vi "Configure SMU.vi"(5 "aperture time":dbl=0.001, 7 "Source Mode":enum16{"Voltage", "Current"}(ring), 8 "error in (no error)":errorcluster, 9 "Settings":T2 {"Sense" items=["Local"=1008, "Remote"=1009]}, 10 "Pins":string[](array[string]), 11 "Semiconductor Module Context":T3) -> (0 "error out":errorcluster)   [LabVIEW 2013]
uses:
  <vilib>/NI_TestStand_SemiconductorModule/NI_TestStand_Semiconductor_Module.lvlibp/PinMap/General/SemiconductorModuleContext.ctl
  <instrlib>/niDCPower/nidcpower.llb/niDCPower Sense.ctl
  <instrlib>/niDCPower/nidcpower.llb/niDCPower Aperture Time Units.ctl
  <instrlib>/niDCPower/nidcpower.llb/niDCPower Output Function.ctl
  <vilib>/NI_TestStand_SemiconductorModule/NI_TestStand_Semiconductor_Module.lvlibp/PinMap/DC Power/PinsToNIDCPowerSessions.vi
  <vilib>/NI_TestStand_SemiconductorModule/NI_TestStand_Semiconductor_Module.lvlibp
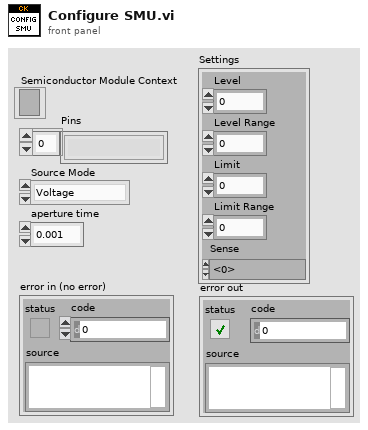
[diagram p1: front panel]
types:
  T1 = typedef "niDCPower Sense.ctl" = i32
  T2 = cluster{"Level":dbl, "Level Range":dbl, "Limit":dbl, "Limit Range":dbl, "Sense":T1}
  T3 = typedef "NI_TestStand_Semiconductor_Module.lvlibp/SemiconductorModuleContext.ctl" = refnum<k7>
  T4 = typedef "niDCPower Aperture Time Units.ctl" = i32
  T5 = typedef "niDCPower Output Function.ctl" = i32
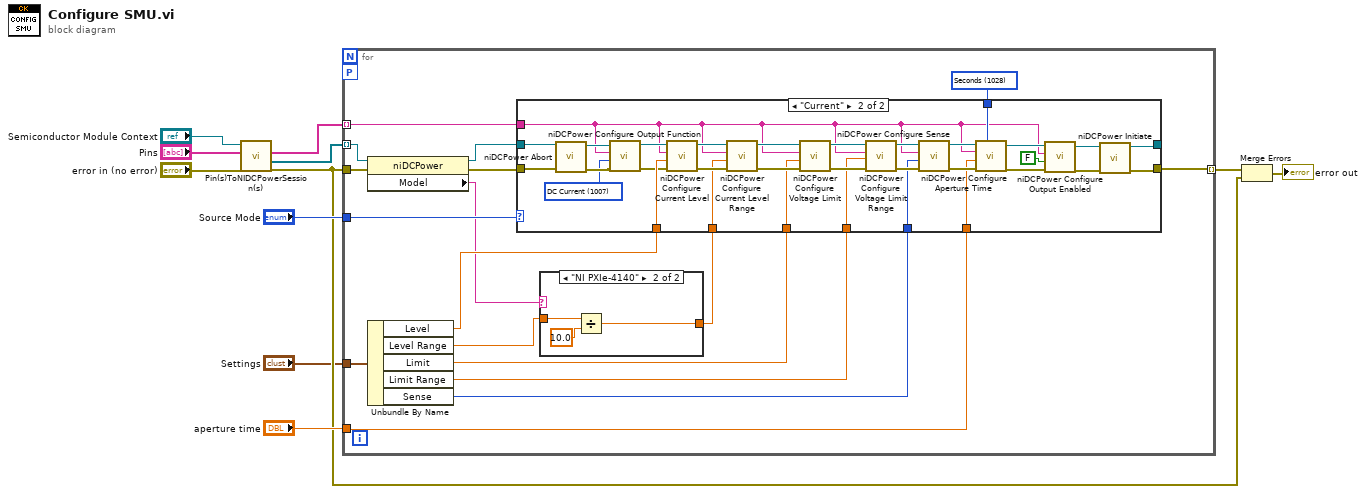
[diagram p0: block diagram]
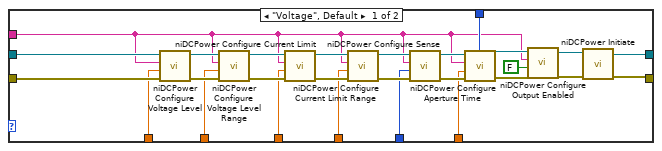
[diagram p3: hidden frame]
diagram:
  n1 = call-poly <vilib>:"Pin(s)ToNIDCPowerSession(s).vi"("error in (no error)"="error in (no error)", "Pins"="Pins", "Semiconductor Module Context"="Semiconductor Module Context") -> ("error out"=w4:errorcluster, "Instrument Sessions"=w9:refnum<k15>[], "Channel Lists"=w8:string[])  [unwired: 4 in, 2 out]
  n2 = for {
    tunnel: w9 -> [w18] mode=indexing
    tunnel: w8 -> [w28] mode=indexing
    tunnel: "Settings" -> [w27]
    tunnel: "Source Mode" -> [w23]
    tunnel: "aperture time" -> [w12]
    tunnel: w4 -> [w19]
    tunnel: [w14] -> w1 mode=indexing
    workers-P: _ -> [_]
    w21 = T4 1028 items=["Seconds"=1028, "Powerline Cycles"=1029] ("aperture time units")
    n3 = property class="niDCPower"(reference=w18, error in=w19) -> (reference out=w17:refnum<k15>, error out=w20:errorcluster, "Model"=w13:string)
    n4 = Unbundle By Name(w27) -> ("Level"=w26:dbl, "Level Range"=w16:dbl, "Limit"=w25:dbl, "Limit Range"=w24:dbl, "Sense"=w22:T1)
    n5 = case shown="\"NI PXIe-4140\"" w13 {
      tunnel: [w29 w30] -> w15
      tunnel: w16 -> [w29 w32]
      frame "NI PXIe-4145", Default {
      }
      frame "NI PXIe-4140" {
        n6 = Divide(x=w32, y=10.0) -> (x/y=w30:dbl)
      }
    }
    n7 = case shown="\"Current\"" w23 {
      tunnel: w20 -> [w59 w74]
      tunnel: w17 -> [w58 w73]
      tunnel: w28 -> [w33 w60]
      tunnel: [w35 w61] -> w14
      tunnel: w26 -> [w49 w91]
      tunnel: w15 -> [w48 w88]
      tunnel: w25 -> [w47 w85]
      tunnel: w24 -> [w46 w82]
      tunnel: w22 -> [w41 w79]
      tunnel: w12 -> [w43 w76]
      tunnel: w21 -> [w42 w75]
      tunnel: [w34 w62] -> _
      frame "Voltage", Default {
        n8 = call <instrlib>:"niDCPower Configure Voltage Level.vi"("error in (no error)"=w59, "voltage level"=w49, "channel name"=w33, "instrument handle"=w58) -> ("error out"=w57:errorcluster, "instrument handle out"=w56:refnum<k15>)  [unwired: 6 in]
        n9 = call <instrlib>:"niDCPower Configure Voltage Level Range.vi"("error in (no error)"=w57, "voltage level range"=w48, "channel name"=w33, "instrument handle"=w56) -> ("error out"=w55:errorcluster, "instrument handle out"=w53:refnum<k15>)  [unwired: 6 in]
        n10 = call <instrlib>:"niDCPower Configure Current Limit.vi"("error in (no error)"=w55, "current limit"=w47, "channel name"=w33, "instrument handle"=w53) -> ("error out"=w54:errorcluster, "instrument handle out"=w52:refnum<k15>)  [unwired: 6 in]
        n11 = call <instrlib>:"niDCPower Configure Current Limit Range.vi"("error in (no error)"=w54, "current limit range"=w46, "channel name"=w33, "instrument handle"=w52) -> ("error out"=w51:errorcluster, "instrument handle out"=w50:refnum<k15>)  [unwired: 6 in]
        n12 = call <instrlib>:"niDCPower Configure Sense.vi"("error in (no error)"=w51, "sense"=w41, "channel name"=w33, "instrument handle"=w50) -> ("error out"=w45:errorcluster, "instrument handle out"=w44:refnum<k15>)  [unwired: 6 in]
        n13 = call <instrlib>:"niDCPower Configure Aperture Time.vi"("aperture time units"=w42, "error in (no error)"=w45, "aperture time"=w43, "channel name"=w33, "instrument handle"=w44) -> ("error out"=w37:errorcluster, "instrument handle out"=w36:refnum<k15>)  [unwired: 5 in]
        n14 = call <instrlib>:"niDCPower Configure Output Enabled.vi"("error in (no error)"=w37, "output enabled"=FALSE, "channel name"=w33, "instrument handle"=w36) -> ("error out"=w39:errorcluster, "instrument handle out"=w40:refnum<k15>)  [unwired: 6 in]
        n15 = call <instrlib>:"niDCPower Initiate.vi"("error in (no error)"=w39, "instrument handle"=w40) -> ("error out"=w35:errorcluster, "instrument handle out"=w34:refnum<k15>)  [unwired: 8 in]
      }
      frame "Current" {
        w68 = T5 1007 items=["DC Voltage"=1006, "DC Current"=1007, "Pulse Voltage"=1049, "Pulse Current"=1050] ("output function")
        n16 = call <instrlib>:"niDCPower Abort.vi"("error in (no error)"=w74, "instrument handle"=w73) -> ("error out"=w70:errorcluster, "instrument handle out"=w69:refnum<k15>)  [unwired: 8 in]
        n17 = call <instrlib>:"niDCPower Configure Output Function.vi"("error in (no error)"=w70, "output function"=w68, "channel name"=w60, "instrument handle"=w69) -> ("error out"=w72:errorcluster, "instrument handle out"=w71:refnum<k15>)  [unwired: 6 in]
        n18 = call <instrlib>:"niDCPower Configure Current Level.vi"("error in (no error)"=w72, "current level"=w91, "channel name"=w60, "instrument handle"=w71) -> ("error out"=w90:errorcluster, "instrument handle out"=w89:refnum<k15>)  [unwired: 6 in]
        n19 = call <instrlib>:"niDCPower Configure Current Level Range.vi"("error in (no error)"=w90, "current level range"=w88, "channel name"=w60, "instrument handle"=w89) -> ("error out"=w87:errorcluster, "instrument handle out"=w86:refnum<k15>)  [unwired: 6 in]
        n20 = call <instrlib>:"niDCPower Configure Voltage Limit.vi"("error in (no error)"=w87, "voltage limit"=w85, "channel name"=w60, "instrument handle"=w86) -> ("error out"=w84:errorcluster, "instrument handle out"=w83:refnum<k15>)  [unwired: 6 in]
        n21 = call <instrlib>:"niDCPower Configure Voltage Limit Range.vi"("error in (no error)"=w84, "voltage limit range"=w82, "channel name"=w60, "instrument handle"=w83) -> ("error out"=w81:errorcluster, "instrument handle out"=w80:refnum<k15>)  [unwired: 6 in]
        n22 = call <instrlib>:"niDCPower Configure Sense.vi"("error in (no error)"=w81, "sense"=w79, "channel name"=w60, "instrument handle"=w80) -> ("error out"=w78:errorcluster, "instrument handle out"=w77:refnum<k15>)  [unwired: 6 in]
        n23 = call <instrlib>:"niDCPower Configure Aperture Time.vi"("aperture time units"=w75, "error in (no error)"=w78, "aperture time"=w76, "channel name"=w60, "instrument handle"=w77) -> ("error out"=w64:errorcluster, "instrument handle out"=w63:refnum<k15>)  [unwired: 5 in]
        n24 = call <instrlib>:"niDCPower Configure Output Enabled.vi"("error in (no error)"=w64, "output enabled"=FALSE, "channel name"=w60, "instrument handle"=w63) -> ("error out"=w66:errorcluster, "instrument handle out"=w65:refnum<k15>)  [unwired: 6 in]
        n25 = call <instrlib>:"niDCPower Initiate.vi"("error in (no error)"=w66, "instrument handle"=w65) -> ("error out"=w61:errorcluster, "instrument handle out"=w62:refnum<k15>)  [unwired: 8 in]
      }
    }
  }
  n26 = Merge Errors(w1, w4) -> (→"error out":errorcluster)
